vi "Test Error.vi"(11 "Dummy In":refnum<class "Example Test Case.lvclass">) -> (0 "error out":errorcluster, 3 "Dummy Out":refnum<class "Example Test Case.lvclass">)   [LabVIEW 2020, in "Example Test Case.lvclass"]
doc: "Test which fails due to an error"
uses:
  Example Test Case.lvclass
  Example Test Case.lvclass/Example Test Case.ctl
  LUnit Test Case.lvclass
  C:/git/astemes-lunit/source/LUnit Test Case.lvclass
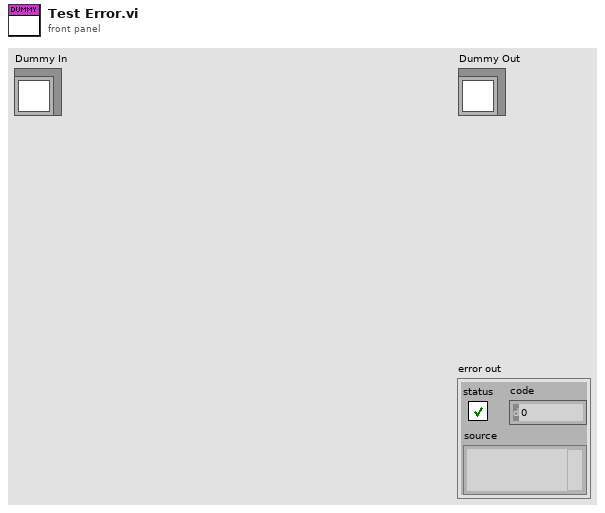
[diagram p1: front panel]
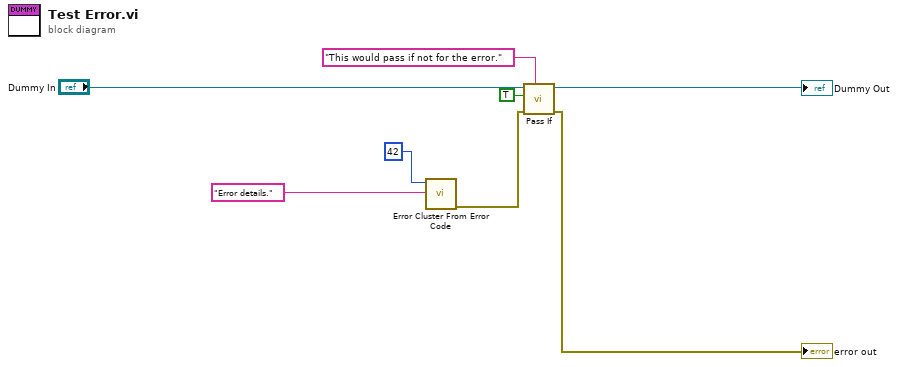
[diagram p0: block diagram]
diagram:
  n1 = call <vilib>:"Error Cluster From Error Code.vi"("error message (\"\")"="Error details." ("Description"), "error code (0)"=42) -> ("error out"=w5:errorcluster)  [unwired: 7 in]
  n2 = call "Pass If.vi"("Description"="This would pass if not for the error.", "error in (no error)"=w5, "Pass?"=TRUE, "LUnit Test Case In"="Dummy In") -> ("error out"=→"error out":errorcluster, "LUnit Test Case Out"=→"Dummy Out":refnum<class "Example Test Case.lvclass">)  [unwired: 6 in]
